vi "Temperature_value_randomizer.vi"() -> (3 "Temperature Value":i32=30)   [LabVIEW 2021]
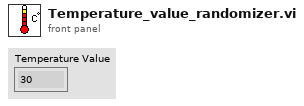
[diagram p1: front panel]
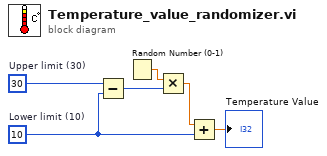
[diagram p0: block diagram]
diagram:
  w2 = 10  # Lower limit (10)
  w5 = 30  # Upper limit (30)
  n1 = Subtract(x=w5, y=w2) -> (x-y=w4:i32)
  n2 = Random Number (0-1)() -> (number: 0 to 1=w6:dbl)
  n3 = Multiply(x=w6, y=w4) -> (x*y=w3:dbl)
  n4 = Add(x=w3, y=w2) -> (x+y=→"Temperature Value":dbl)
